vi "Button Toggle Motor.vi"(6 "Control Mode":T1 items=["PercentOutput"=0, "Position"=1, "Velocity"=2, "Current"=3, "Follower"=5, "MotionProfile"=6, "MotionMagic"=7, "MotionMagicArc"=8, "MotionProfileArc"=10, "Disabled"=15], 8 "error in (no error)":errorcluster, 9 "Motor Power":dbl format="%#_13g", 10 "refnum name":string="My Motor RefNum", 11 "Input":bool) -> (0 "error out":errorcluster)   [LabVIEW 2017, in "Huskie Swerve.lvlib"]
uses:
  Huskie Swerve.lvlib
  <vilib>/Rock Robotics/WPI/ThirdParty/Phoenix-LabVIEW/Motor Controller/Controls/CTRE_Phoenix_MotorControl_ControlMode.ctl
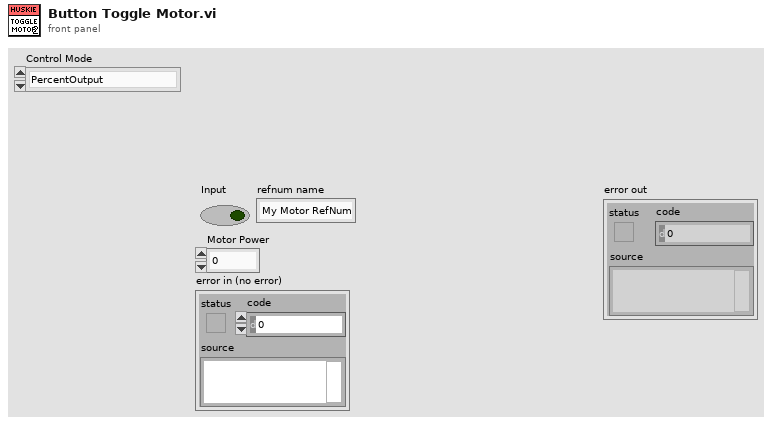
[diagram p1: front panel]
types:
  T1 = typedef "CTRE_Phoenix_MotorControl_ControlMode.ctl" = u16
  T2 = typedef "WPI_MotorControlDeviceRef.ctl" = cluster{"DeviceStatus":errorcluster, "Type":T3, "PWM":cluster{"PWM Channel":T4, "DeadBand":T5}, "CAN":cluster{"Device Number":u8, "SetOutput VI Ref":variant, "GetOutput VI Ref":variant, "Enable VI Ref":variant, "Disable VI Ref":variant, "Data":variant}, "Invert":bool, "DIO PWM":cluster{"PWM \"Enable\" Channel":T4, "DIOChannel":T6, "PWM Rate":dbl}}
  T3 = typedef "WPI_MotorControlType.ctl" = enum16{"PWM", "CAN", "DIO PWM"}
  T4 = typedef "FPGA_DIOPWMChannel.ctl" = enum8{"PWM 0", "PWM 1", "PWM 2", "PWM 3", "PWM 4", "PWM 5", "PWM 6", "PWM 7", "PWM 8", "PWM 9", "PWM MXP 0", "PWM MXP 1", "PWM MXP 2", "PWM MXP 3", "PWM MXP 4", "PWM MXP 5", "PWM MXP 6", "PWM MXP 7", "PWM MXP 8", "PWM MXP 9", "Invalid"}
  T5 = typedef "WPI_PWMDeadband.ctl" = cluster{"Name":string, "maxPositivePwm":i32, "minPositivePwm":i32, "centerPwm":i32, "maxNegativePwm":i32, "minNegativePwm":i32, "angularRange":u16}
  T6 = typedef "FPGA_DIOChannel.ctl" = enum8{"DIO 0", "DIO 1", "DIO 2", "DIO 3", "DIO 4", "DIO 5", "DIO 6", "DIO 7", "DIO 8", "DIO 9", "DIO MXP 0", "DIO MXP 1", "DIO MXP 2", "DIO MXP 3", "DIO MXP 4", "DIO MXP 5", "DIO MXP 6", "DIO MXP 7", "DIO MXP 8", "DIO MXP 9", "DIO MXP 10", "DIO MXP 11", "DIO MXP 12", "DIO MXP 13", "DIO MXP 14", "DIO MXP 15", "SPI Port CS1", "SPI Port CS2", "SPI Port CS3", "SPI Port MISO", "SPI Port MOSI", "Invalid"}
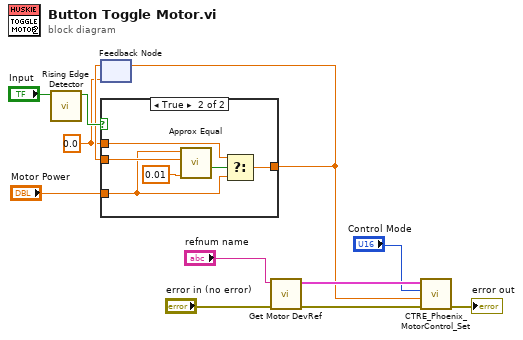
[diagram p0: block diagram]
diagram:
  w6 = 0.0 ("f")
  n1 = call "Rising Edge Detector.vi"("Input"="Input") -> ("Rising edge?"=w9:bool)  [unwired: 10 in]
  n2 = feedback #1(w6) -> (w8:dbl)
  n3 = case shown="True" w9 {
    tunnel: w8 -> [w13 w19]
    tunnel: "Motor Power" -> [_ w15]
    tunnel: w6 -> [_ w16]
    tunnel: [w13 w14] -> w4
    frame False {
    }
    frame True {
      n4 = call "Approx Equal.vi"("Tolerance"=0.01, "b"=w19, "a"=w15) -> ("a == b?"=w17:bool)  [unwired: 8 in]
      n5 = Select(t=w16, s=w17, f=w15) -> (s? t:f=w14:dbl)
    }
  }
  n6 = feedback-in #1(w4) -> ()
  n7 = call "Get Motor DevRef.vi"("error in (no error)"="error in (no error)", "refnum name"="refnum name") -> ("error out"=w3:errorcluster, "PhoenixMotorControlDevRef"=w5:T2)  [unwired: 8 in]
  n8 = call "CTRE_Phoenix_MotorControl_Set.vi"("error in (no error)"=w3, "Output"=w4, "Control Mode"="Control Mode", "PhoenixMotorControlDevRef"=w5) -> ("error out"=→"error out":errorcluster)  [unwired: 6 in, 1 out]
